vi "Name.vi"(8 "error in (no error)":errorcluster, 11 "VolatusConfigElement in":refnum<class "VolatusConfigElement.lvclass">) -> (0 "error out":errorcluster, 2 "Name":string, 3 "VolatusConfigElement out":refnum<class "VolatusConfigElement.lvclass">)   [LabVIEW 2020, in "VolatusConfig.lvlib" / "VolatusConfigElement.lvclass"]
uses:
  VolatusConfigElement.lvclass
  VolatusConfigElement.lvclass/VolatusConfigElement.ctl
  lv-cdm/CDM-Config/Config Element/Config Element.lvclass
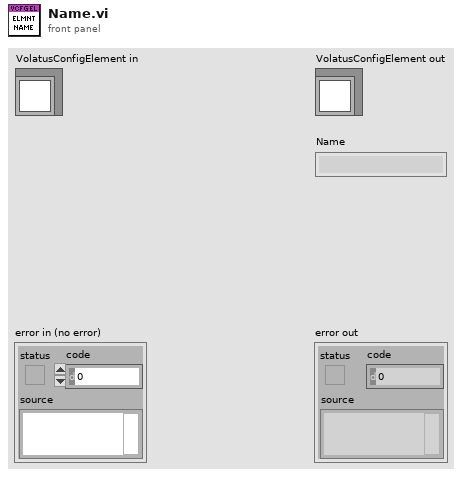
[diagram p1: front panel]
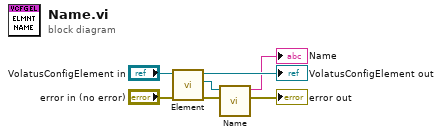
[diagram p0: block diagram]
diagram:
  n1 = call "Element.vi"("VolatusConfigElement in"="VolatusConfigElement in") -> ("Element"=w2:refnum<class "Config Element.lvclass">, "VolatusConfigElement out"=→"VolatusConfigElement out":refnum<class "VolatusConfigElement.lvclass">)  [unwired: 9 in]
  n2 = call "Name.vi"("error in (no error)"="error in (no error)", "Config Element in"=w2) -> ("Name"=→"Name":string)  [unwired: 8 in, 1 out]
  "error out" <- "error in (no error)"
